vi "global_qaqc.vi"() -> ()   [LabVIEW 2015]
panel:
  out "String":string
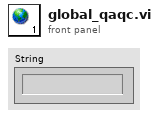
[diagram p1: front panel]
diagram:
